vi "UserID.vi"(10 "User Index in":i32) -> (0 "valid user":bool caption="Usuario Válido", 1 "User Information out":T1 caption="Informacion del Usario" {"Country" items=["Afghanistan", "Aland Islands", "Albania", "Algeria", "American Samoa", "Andorra", "Angola", "Anguilla", "Antarctica", "Antigua And Barbuda", "Argentina", "Armenia", "Aruba", "Australia", "Austria", "Azerbaijan", "Bahamas", "Bahrain", "Bangladesh", "Barbados", "Belarus", "Belgium", "Belize", "Benin", "Bermuda", "Bhutan", "Bolivia", "Bosnia And Herzegovina", "Botswana", "Bouvet Island", "Brazil", "British Indian Ocean Territory", "Brunei Darussalam", "Bulgaria", "Burkina Faso", "Burundi", "Cambodia", "Cameroon", "Canada", "Cape Verde", "Cayman Islands", "Central African Republic", "Chad", "Chile", "China", "Christmas Island", "Cocos (Keeling) Islands", "Colombia", "Comoros", "Congo", "Congo, The Democratic Republic Of The", "Cook Islands", "Costa Rica", "Cote D'Ivoire", "Croatia", "Cuba", "Cyprus", "Czech Republic", "Denmark", "Djibouti", "Dominica", "Dominican Republic", "Ecuador", "Egypt", "El Salvador", "Equatorial Guinea", "Eritrea", "Estonia", "Ethiopia", "Falkland Islands (Malvinas)", "Faroe Islands", "Fiji", "Finland", "France", "French Guiana", "French Polynesia", "French Southern Territories", "Gabon", "Gambia", "Georgia", "Germany", "Ghana", "Gibraltar", "Greece", "Greenland", "Grenada", "Guadeloupe", "Guam", "Guatemala", "Guernsey", "Guinea", "Guinea-Bissau", "Guyana", "Haiti", "Heard Island And Mcdonald Islands", "Holy See (Vatican City State)", "Honduras", "Hong Kong", "Hungary", "Iceland", "India", "Indonesia", "Iran, Islamic Republic Of", "Iraq", "Ireland", "Isle Of Man", "Israel", "Italy", "Jamaica", "Japan", "Jersey", "Jordan", "Kazakhstan", "Kenya", "Kiribati", "Korea, Democratic People'S Republic Of", "Korea, Republic Of", "Kuwait", "Kyrgyzstan", "Lao People'S Democratic Republic", "Latvia", "Lebanon", "Lesotho", "Liberia", "Libyan Arab Jamahiriya", "Liechtenstein", "Lithuania", "Luxembourg", "Macao", "Macedonia, The Former Yugoslav Republic Of", "Madagascar", "Malawi", "Malaysia", "Maldives", "Mali", "Malta", "Marshall Islands", "Martinique", "Mauritania", "Mauritius", "Mayotte", "Mexico", "Micronesia, Federated States Of", "Moldova, Republic Of", "Monaco", "Mongolia", "Montserrat", "Morocco", "Mozambique", "Myanmar", "Namibia", "Nauru", "Nepal", "Netherlands", "Netherlands Antilles", "New Caledonia", "New Zealand", "Nicaragua", "Niger", "Nigeria", "Niue", "Norfolk Island", "Northern Mariana Islands", "Norway", "Oman", "Pakistan", "Palau", "Palestinian Territory, Occupied", "Panama", "Papua New Guinea", "Paraguay", "Peru", "Philippines", "Pitcairn", "Poland", "Portugal", "Puerto Rico", "Qatar", "Reunion", "Romania", "Russian Federation", "Rwanda", "Saint Helena", "Saint Kitts And Nevis", "Saint Lucia", "Saint Pierre And Miquelon", "Saint Vincent And The Grenadines", "Samoa", "San Marino", "Sao Tome And Principe", "Saudi Arabia", "Senegal", "Serbia And Montenegro", "Seychelles", "Sierra Leone", "Singapore", "Slovakia", "Slovenia", "Solomon Islands", "Somalia", "South Africa", "South Georgia And The South Sandwich Islands", "Spain", "Sri Lanka", "Sudan", "Suriname", "Svalbard And Jan Mayen", "Swaziland", "Sweden", "Switzerland", "Syrian Arab Republic", "Taiwan, Province Of China", "Tajikistan", "Tanzania, United Republic Of", "Thailand", "Timor-Leste", "Togo", "Tokelau", "Tonga", "Trinidad And Tobago", "Tunisia", "Turkey", "Turkmenistan", "Turks And Caicos Islands", "Tuvalu", "Uganda", "Ukraine", "United Arab Emirates", "United Kingdom", "United States", "United States Minor Outlying Islands", "Uruguay", "Uzbekistan", "Vanuatu", "Venezuela", "Viet Nam", "Virgin Islands, British", "Virgin Islands, U.S.", "Wallis And Futuna", "Western Sahara", "Yemen", "Zambia", "Zimbabwe", "(Not Specified)"]}, 2 "User Index out":i32)   [LabVIEW 2015, in "AguaClara Library.lvlib"]
uses:
  AguaClara Library.lvlib
  User status cmd.ctl
  User status.ctl
  Register options.ctl
  User Information.ctl
  Country Ring.ctl
panel:
  in  "Cancel Button":bool caption="Cancelar"
  in  "User Information":T1 caption="Informacion del usario" {"Country" items=["Afghanistan", "Aland Islands", "Albania", "Algeria", "American Samoa", "Andorra", "Angola", "Anguilla", "Antarctica", "Antigua And Barbuda", "Argentina", "Armenia", "Aruba", "Australia", "Austria", "Azerbaijan", "Bahamas", "Bahrain", "Bangladesh", "Barbados", "Belarus", "Belgium", "Belize", "Benin", "Bermuda", "Bhutan", "Bolivia", "Bosnia And Herzegovina", "Botswana", "Bouvet Island", "Brazil", "British Indian Ocean Territory", "Brunei Darussalam", "Bulgaria", "Burkina Faso", "Burundi", "Cambodia", "Cameroon", "Canada", "Cape Verde", "Cayman Islands", "Central African Republic", "Chad", "Chile", "China", "Christmas Island", "Cocos (Keeling) Islands", "Colombia", "Comoros", "Congo", "Congo, The Democratic Republic Of The", "Cook Islands", "Costa Rica", "Cote D'Ivoire", "Croatia", "Cuba", "Cyprus", "Czech Republic", "Denmark", "Djibouti", "Dominica", "Dominican Republic", "Ecuador", "Egypt", "El Salvador", "Equatorial Guinea", "Eritrea", "Estonia", "Ethiopia", "Falkland Islands (Malvinas)", "Faroe Islands", "Fiji", "Finland", "France", "French Guiana", "French Polynesia", "French Southern Territories", "Gabon", "Gambia", "Georgia", "Germany", "Ghana", "Gibraltar", "Greece", "Greenland", "Grenada", "Guadeloupe", "Guam", "Guatemala", "Guernsey", "Guinea", "Guinea-Bissau", "Guyana", "Haiti", "Heard Island And Mcdonald Islands", "Holy See (Vatican City State)", "Honduras", "Hong Kong", "Hungary", "Iceland", "India", "Indonesia", "Iran, Islamic Republic Of", "Iraq", "Ireland", "Isle Of Man", "Israel", "Italy", "Jamaica", "Japan", "Jersey", "Jordan", "Kazakhstan", "Kenya", "Kiribati", "Korea, Democratic People'S Republic Of", "Korea, Republic Of", "Kuwait", "Kyrgyzstan", "Lao People'S Democratic Republic", "Latvia", "Lebanon", "Lesotho", "Liberia", "Libyan Arab Jamahiriya", "Liechtenstein", "Lithuania", "Luxembourg", "Macao", "Macedonia, The Former Yugoslav Republic Of", "Madagascar", "Malawi", "Malaysia", "Maldives", "Mali", "Malta", "Marshall Islands", "Martinique", "Mauritania", "Mauritius", "Mayotte", "Mexico", "Micronesia, Federated States Of", "Moldova, Republic Of", "Monaco", "Mongolia", "Montserrat", "Morocco", "Mozambique", "Myanmar", "Namibia", "Nauru", "Nepal", "Netherlands", "Netherlands Antilles", "New Caledonia", "New Zealand", "Nicaragua", "Niger", "Nigeria", "Niue", "Norfolk Island", "Northern Mariana Islands", "Norway", "Oman", "Pakistan", "Palau", "Palestinian Territory, Occupied", "Panama", "Papua New Guinea", "Paraguay", "Peru", "Philippines", "Pitcairn", "Poland", "Portugal", "Puerto Rico", "Qatar", "Reunion", "Romania", "Russian Federation", "Rwanda", "Saint Helena", "Saint Kitts And Nevis", "Saint Lucia", "Saint Pierre And Miquelon", "Saint Vincent And The Grenadines", "Samoa", "San Marino", "Sao Tome And Principe", "Saudi Arabia", "Senegal", "Serbia And Montenegro", "Seychelles", "Sierra Leone", "Singapore", "Slovakia", "Slovenia", "Solomon Islands", "Somalia", "South Africa", "South Georgia And The South Sandwich Islands", "Spain", "Sri Lanka", "Sudan", "Suriname", "Svalbard And Jan Mayen", "Swaziland", "Sweden", "Switzerland", "Syrian Arab Republic", "Taiwan, Province Of China", "Tajikistan", "Tanzania, United Republic Of", "Thailand", "Timor-Leste", "Togo", "Tokelau", "Tonga", "Trinidad And Tobago", "Tunisia", "Turkey", "Turkmenistan", "Turks And Caicos Islands", "Tuvalu", "Uganda", "Ukraine", "United Arab Emirates", "United Kingdom", "United States", "United States Minor Outlying Islands", "Uruguay", "Uzbekistan", "Vanuatu", "Venezuela", "Viet Nam", "Virgin Islands, British", "Virgin Islands, U.S.", "Wallis And Futuna", "Western Sahara", "Yemen", "Zambia", "Zimbabwe", "(Not Specified)"]}
  out "logon status":T3=enum."unregistered email" caption="Log on Status"
  in  "Okay Button":bool caption="OK"
  in  "Valid User Options":T4 caption="Lista de Opciones validas"
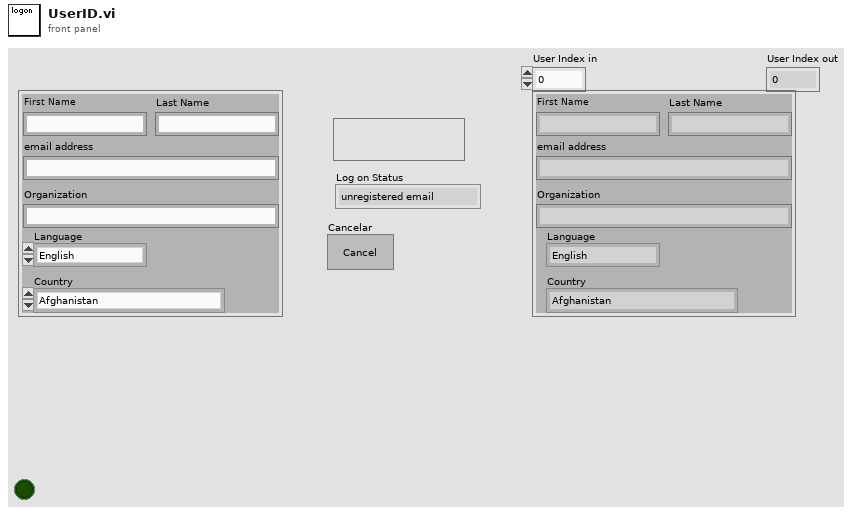
[diagram p1: front panel]
types:
  T1 = typedef "AguaClara Library.lvlib/User Information.ctl" = cluster{"First Name":string, "Last Name":string, "Email Address":string, "Organization":string, "Language":enum16{"English", "Español", "French"}, "Country":T2}
  T2 = typedef "Country Ring.ctl" = u16
  T3 = typedef "AguaClara Library.lvlib/User status.ctl" = enum16{"invalid email", "unregistered email", "registered email"}
  T4 = typedef "AguaClara Library.lvlib/Register options.ctl" = cluster{"New Account":bool, "Update User Info":bool}
  T5 = typedef "AguaClara Library.lvlib/User status cmd.ctl" = enum16{"Load File Path", "Create account", "Update user", "Email password", "Load inputs", "Check status"}
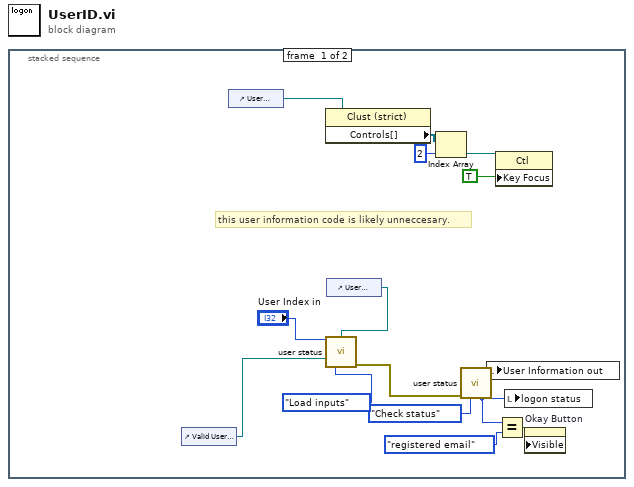
[diagram p0: block diagram]
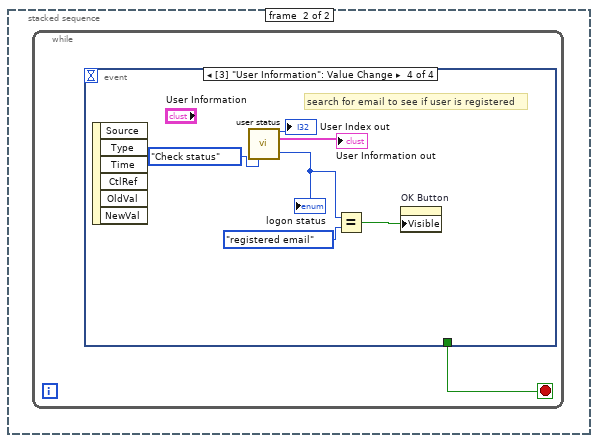
[diagram p2: hidden frame]
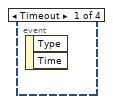
[diagram p3: hidden frame]
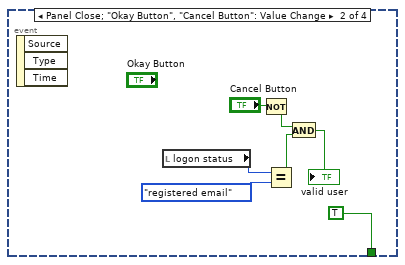
[diagram p4: hidden frame]
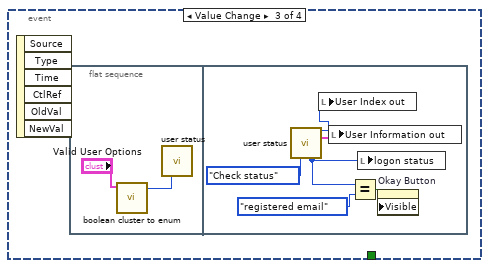
[diagram p5: hidden frame]
diagram:
  n1 = stacked-sequence {
    frame #0 {
      # "this user information code is likely unneccesary."
      n2 = control-ref of="Valid User Options"() -> (w9:refnum<vi>)
      n3 = control-ref of="User Information"() -> (w14:refnum<vi>)
      n4 = property class="Clust (strict)"(reference=w14) -> ("Controls[]"=w10:refnum<vi>[])  [unwired: 1 in, 2 out]
      n5 = control-ref of="User Information"() -> (w1:refnum<vi>)
      n6 = call "user status.vi"("User Index in"="User Index in", "User Info"=w1, "User Options"=w9, "User status cmd"=User_status_cmd."Load inputs") -> ("error out"=w2:errorcluster)  [unwired: 7 in, 4 out]
      n7 = Index Array(array=w10, index=2) -> (element=w12:refnum<vi>)
      n8 = call "user status.vi"("error in (no error)"=w2, "User status cmd"=User_status_cmd."Check status") -> ("User Information out"=w3:T1, "logon status"=w7:T3)  [unwired: 9 in, 3 out]
      n9 = local write "User Information out"(w3) -> ()
      n10 = property class="Ctl"(reference=w12, "Key Focus"=TRUE) -> ()  [unwired: 1 in, 2 out]
      n11 = Equal?(x=w7, y=User_status."registered email" ("logon status")) -> (x = y?=w5:bool)
      n12 = local write "logon status"(w7) -> ()
      n13 = property on="Okay Button" class="Bool"("Visible"=w5) -> ()  [unwired: 2 in, 2 out]
    }
    frame #1 {
      n14 = while {
        stop <- w16 stop-if-true
        n15 = event shown="[3] \"User Information\": Value Change" {
          selector: _ -> [_ _ _ _]
          dyn-events: _ -> [_ _ _ _]
          timeout: _ -> [_ _ _ _]
          tunnel: [_ TRUE _ _] -> w16
          event Timeout {
            n16 = event-data() -> ()  [unwired: 1 in, 2 out]
          }
          event Panel Close; "Okay Button", "Cancel Button": Value Change {
            n17 = event-data() -> ()  [unwired: 1 in, 3 out]
            n18 = local read "logon status"() -> (w22:T3)
            n19 = Not(x="Cancel Button") -> (.not. x?=w18:bool)
            n20 = Equal?(x=w22, y=User_status."registered email" ("logon status")) -> (x = y?=w20:bool)
            n21 = And(x=w18, y=w20) -> (x .and. y?=→"valid user":bool)
          }
          event Value Change {
            n22 = event-data() -> ()  [unwired: 1 in, 6 out]
            n23 = flat-sequence {
              frame #0 {
                n24 = call "boolean cluster to enum.vi"("Valid User Options"="Valid User Options") -> ("User Options"=w24:T5)  [unwired: 10 in]
                n25 = call "user status.vi"("User status cmd"=w24) -> ()  [unwired: 10 in, 5 out]
              }
              frame #1 {
                n26 = call "user status.vi"("User status cmd"=User_status_cmd."Check status") -> ("User Index"=w26:i32, "User Information out"=w27:T1, "logon status"=w31:T3)  [unwired: 10 in, 2 out]
                n27 = local write "User Index out"(w26) -> ()
                n28 = local write "User Information out"(w27) -> ()
                n29 = Equal?(x=w31, y=User_status."registered email" ("logon status")) -> (x = y?=w29:bool)
                n30 = local write "logon status"(w31) -> ()
                n31 = property on="Okay Button" class="Bool"("Visible"=w29) -> ()  [unwired: 2 in, 2 out]
              }
            }
          }
          event Value Change {
            # "search for email to see if user is registered"
            n32 = event-data() -> ()  [unwired: 1 in, 6 out]
            n33 = call "user status.vi"("User status cmd"=User_status_cmd."Check status") -> ("User Index"=→"User Index out":i32, "User Information out"=→"User Information out":T1, "logon status"=w35:T3)  [unwired: 10 in, 2 out]
            "logon status" <- w35
            n34 = Equal?(x=w35, y=User_status."registered email" ("logon status")) -> (x = y?=w33:bool)
            n35 = property on="OK Button" class="Bool"("Visible"=w33) -> ()  [unwired: 2 in, 2 out]
          }
        }
      }
    }
  }
